vi "S2C_STEP_ShowSettings.vi"(7 "Error In":errorcluster, 10 "Row":i32, 11 "Data In":string[][](array[string])) -> (3 "Data Out":string[][](array[string]), 5 "Error Out":errorcluster)   [LabVIEW 2015]
panel:
  out "Init":bool
  in  "StepName":string="<Enter Name for Step>" caption="Step Name"
  in  "Done":bool
  in  "Settings":i32(listbox) caption="Step Settings"
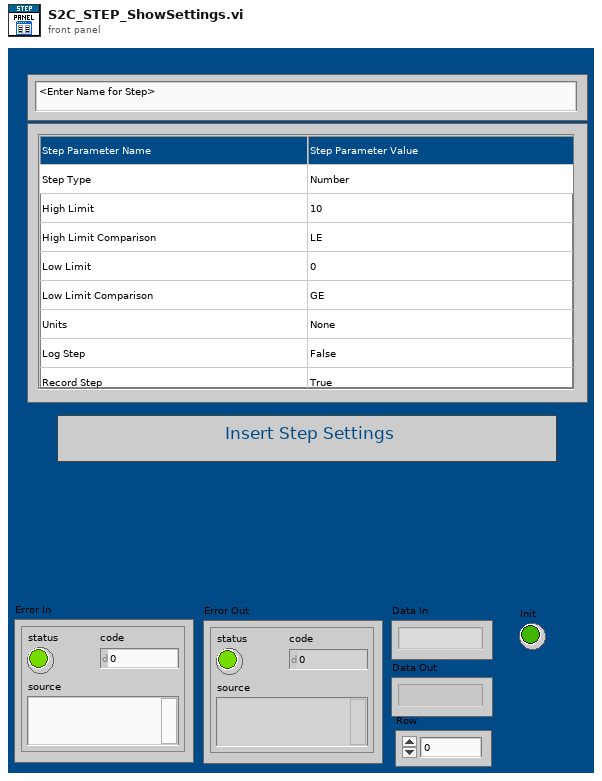
[diagram p1: front panel]
types:
  T1 = cluster{"Selection Start":u32, "Selection End":u32}
  T2 = typedef "LVPoint32TypeDef.ctl" = cluster{"Horizontal":i32, "Vertical":i32}
  T3 = typedef "LVRowAndColumnTypeDef.ctl" = cluster{"Row":i32, "Column":i32}
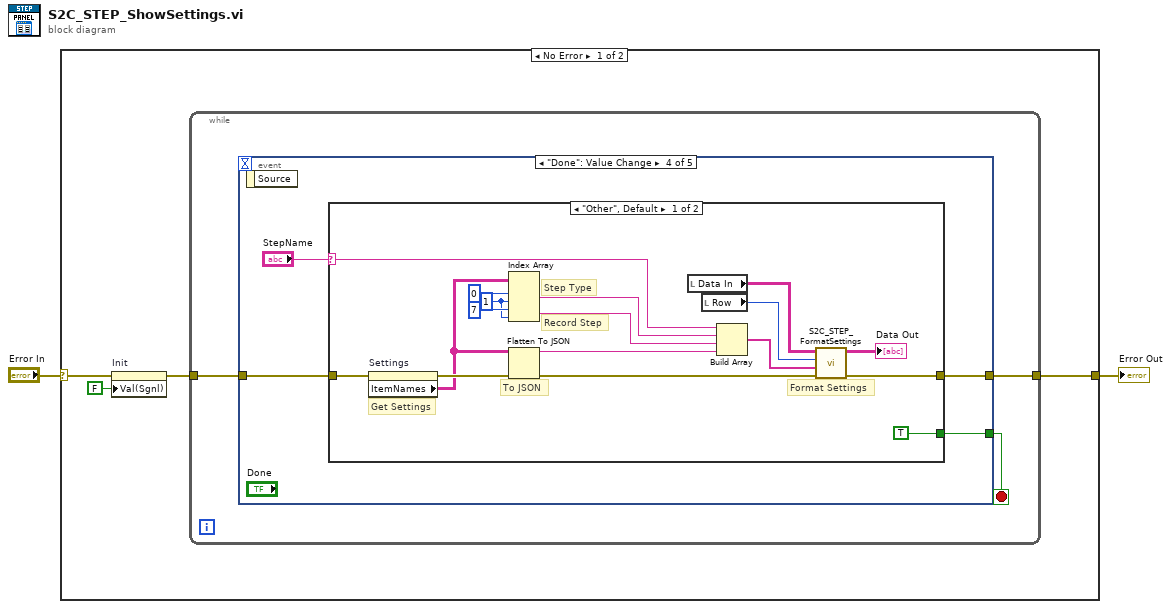
[diagram p0: block diagram]
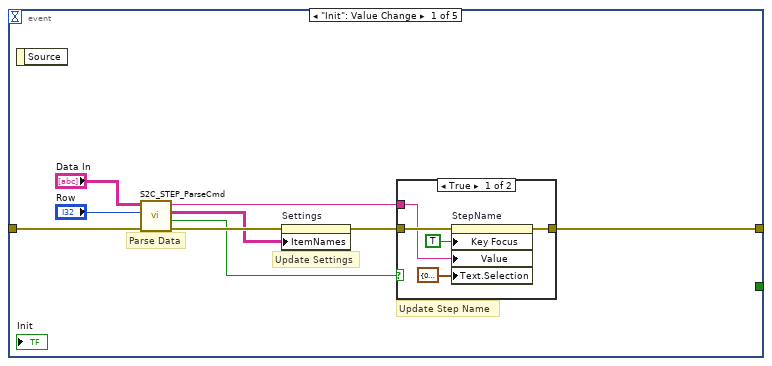
[diagram p2: hidden frame]
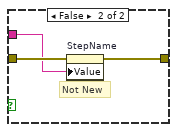
[diagram p3: hidden frame]
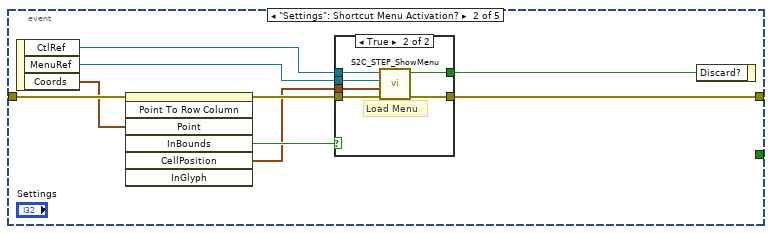
[diagram p4: hidden frame]
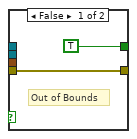
[diagram p5: hidden frame]
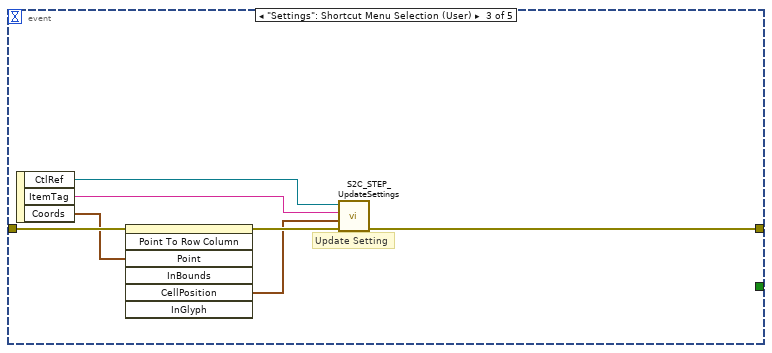
[diagram p6: hidden frame]
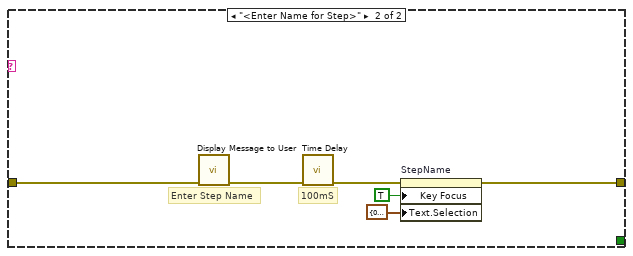
[diagram p7: hidden frame]
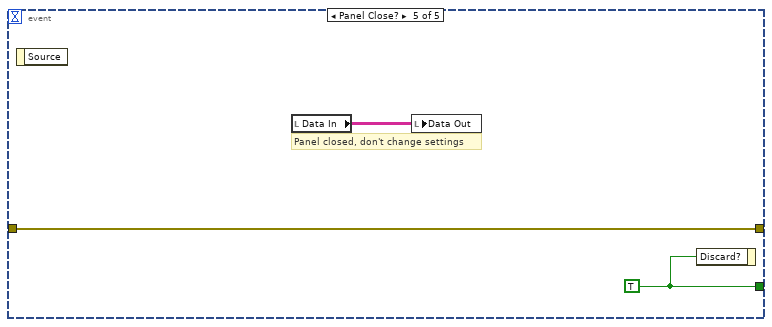
[diagram p8: hidden frame]
diagram:
  n1 = case shown="No Error" "Error In" {
    selector: "Error In" -> [w4 w81]
    tunnel: [w6 w81] -> w1
    frame No Error {
      n2 = property on="Init" class="Bool (strict)"(error in=w4, "Val(Sgnl)"=FALSE ("Value (Signaling)")) -> (error out=w3:errorcluster)  [unwired: 1 in, 1 out]
      n3 = while {
        tunnel: w3 -> [w7]
        tunnel: [w9] -> w6
        stop <- w8 stop-if-true
        n4 = event shown="[3] \"Done\": Value Change" {
          selector: _ -> [_ _ _ _ _]
          dyn-events: _ -> [_ _ _ _ _]
          timeout: _ -> [_ _ _ _ _]
          tunnel: w7 -> [w10 w35 w47 w53 w79]
          tunnel: [w11 w30 w50 w52 w79] -> w9
          tunnel: [_ _ _ w54 w78] -> w8
          event "Init": Value Change {
            # "Update Settings"
            # "Update Step Name"
            # "Parse Data"
            n5 = event-data() -> ()  [unwired: 1 in, 1 out]
            n6 = call "S2C_STEP_ParseCmd.vi"("Error In"=w10, "Row"="Row", "Data In"="Data In") -> ("Error Out"=w16:errorcluster, "New?"=w12:bool, "Settings"=w15:string[][], "Step Name"=w13:string)  [unwired: 5 in]
            n7 = property on="Settings" class="MCListbox (strict)"(error in=w16, "ItemNames"=w15) -> (error out=w14:errorcluster)  [unwired: 1 in, 1 out]
            n8 = case shown="True" w12 {
              tunnel: w14 -> [w21 w26]
              tunnel: w13 -> [w20 w24]
              tunnel: [w19 w25] -> w11
              frame True {
                n9 = property on="StepName" class="Str"(error in=w21, "Key Focus"=TRUE, "Value"=w20, "Text.Selection"=T1 {"Selection Start"=0, "Selection End"=21}) -> (error out=w19:errorcluster)  [unwired: 1 in, 1 out]
              }
              frame False {
                # "Not New"
                n10 = property on="StepName" class="Str"(error in=w26, "Value"=w24) -> (error out=w25:errorcluster)  [unwired: 1 in, 1 out]
              }
            }
          }
          event "Settings": Shortcut Menu Activation? {
            n11 = event-data() -> ("CtlRef"=w28:refnum<vi>, "MenuRef"=w27:refnum<k9>, "Coords"=w34:T2)  [unwired: 1 in]
            n12 = invoke on="Settings" class="MCListbox (strict)" method="Point To Row Column"(error in=w35, "Point"=w34) -> (error out=w33:errorcluster, "InBounds"=w32:bool, "CellPosition"=w31:T3)  [unwired: 5 in, 4 out]
            n13 = case shown="True" w32 {
              tunnel: w33 -> [w37 w43]
              tunnel: w31 -> [_ w40]
              tunnel: w28 -> [_ w42]
              tunnel: [w37 w39] -> w30
              tunnel: [TRUE w38] -> w29
              tunnel: w27 -> [_ w41]
              frame False {
                # "Out of Bounds"
              }
              frame True {
                # "Load Menu"
                n14 = call "S2C_STEP_ShowMenu.vi"("Error In"=w43, "Cell Position"=w40, "MenuRef"=w41, "CtlRef"=w42) -> ("Error Out"=w39:errorcluster, "Discard?"=w38:bool)  [unwired: 6 in]
              }
            }
            n15 = event-data("Discard?"=w29) -> ()  [unwired: 1 in, 1 out]
          }
          event "Settings": Shortcut Menu Selection (User) {
            # "Update Setting"
            n16 = event-data() -> ("CtlRef"=w48:refnum<vi>, "ItemTag"=w49:string, "Coords"=w46:T2)  [unwired: 1 in]
            n17 = invoke on="Settings" class="MCListbox (strict)" method="Point To Row Column"(error in=w47, "Point"=w46) -> (error out=w45:errorcluster, "CellPosition"=w44:T3)  [unwired: 5 in, 5 out]
            n18 = call "S2C_STEP_UpdateSettings.vi"("Error In"=w45, "Cell Position"=w44, "ItemTag"=w49, "CtlRef"=w48) -> ("Error Out"=w50:errorcluster)  [unwired: 7 in]
          }
          event "Done": Value Change {
            n19 = event-data() -> ()  [unwired: 1 in, 1 out]
            n20 = case shown="\"Other\", Default" "StepName" {
              selector: "StepName" -> [w58 _]
              tunnel: [TRUE _] -> w54
              tunnel: w53 -> [w70 w77]
              tunnel: [w63 w74] -> w52
              frame "Other", Default {
                w56 = 1 ("disabled index (col)")
                # "Record Step"
                # "Format Settings"
                # "Step Type"
                # "Get Settings"
                # "To JSON"
                n21 = property on="Settings" class="MCListbox (strict)"(error in=w70) -> (error out=w68:errorcluster, "ItemNames"=w67:string[][])  [unwired: 1 in, 1 out]
                n22 = Index Array(array=w67, index (row) #1=0 ("index (row)"), index (col) #1=w56, index (row) #2=7 ("index (col)"), index (col) #2=w56) -> (element #1=w61:string, element #2=w55:string)
                n23 = Flatten To JSON(anything=w67, error in (no error)=w68) -> (JSON string=w62:string, 11:w66:errorcluster)  [unwired: 1 in]
                n24 = local read "Data In"() -> (w59:string[][])
                n25 = local read "Row"() -> (w60:i32)
                n26 = Build Array(w58, w61, w55, w62) -> (w65:string[])
                n27 = call "S2C_STEP_FormatSettings.vi"("Error In"=w66, "Settings"=w65, "Row"=w60, "Data In"=w59) -> ("Error Out"=w63:errorcluster, "Data Out"=→"Data Out":string[][])  [unwired: 6 in]
              }
              frame "<Enter Name for Step>" {
                # "100mS"
                # "Enter Step Name"
                n28 = call "Display Message to User"("error in (no error)"=w77) -> ("error out"=w73:errorcluster)  [unwired: 9 in, 1 out]
                n29 = call "Time Delay"("error in (no error)"=w73) -> ("error out"=w72:errorcluster)  [unwired: 10 in]
                n30 = property on="StepName" class="Str"(error in=w72, "Key Focus"=TRUE, "Text.Selection"=T1 {"Selection Start"=0, "Selection End"=21}) -> (error out=w74:errorcluster)  [unwired: 1 in, 1 out]
              }
            }
          }
          event Panel Close? {
            w78 = TRUE ("Discard?")
            # "Panel closed, don't change settings"
            n31 = event-data() -> ()  [unwired: 1 in, 1 out]
            n32 = local read "Data In"() -> (w80:string[][])
            n33 = local write "Data Out"(w80) -> ()
            n34 = event-data("Discard?"=w78) -> ()  [unwired: 1 in, 1 out]
          }
        }
      }
    }
    frame Error {
    }
  }
  "Error Out" <- w1
